vi "Set Motor Outputs.vi"(11 "Updated Drive Metrics in":T1) -> (3 "Updated Drive Metrics out":T1)   [LabVIEW 2014]
uses:
  Drive Train Metrics.ctl
  CmdFlag.ctl
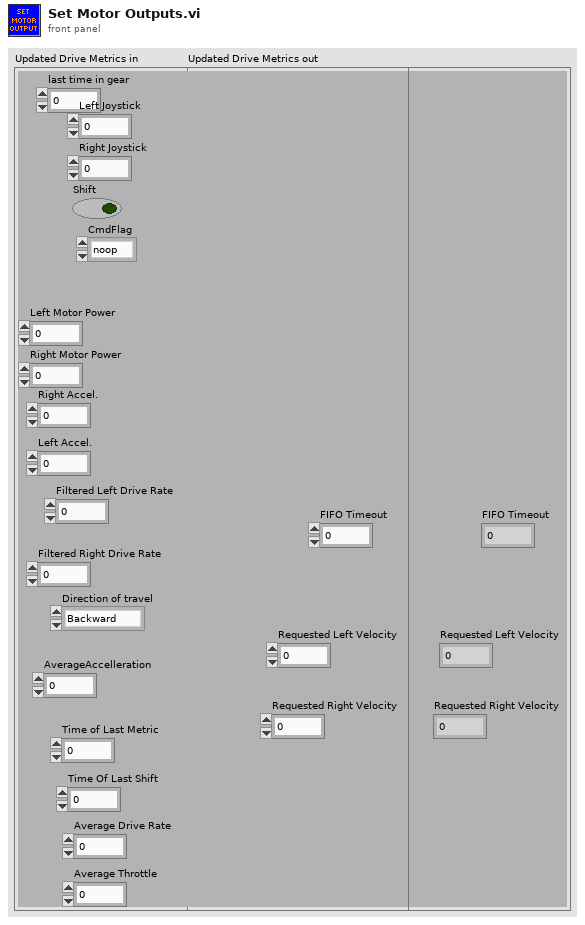
[diagram p1: front panel]
types:
  T1 = typedef "Drive Train Metrics.ctl" = cluster{"last time in gear":u32, "Shift":bool, "Right Joystick":dbl, "Left Joystick":dbl, "CmdFlag":T2, "Right Motor Power":dbl, "Left Motor Power":dbl, "Right Accel.":dbl, "Left Accel.":dbl, "Filtered Left Drive Rate":dbl, "Filtered Right Drive Rate":dbl, "Direction of travel":enum16{"Backward", "Forward", "Spin"}, "AverageAccelleration":dbl, "Time of Last Metric":u32, "Time Of Last Shift":dbl, "Average Drive Rate":dbl, "Average Throttle":dbl, "FIFO Timeout":i32, "Requested Left Velocity":dbl, "Requested Right Velocity":dbl}
  T2 = typedef "CmdFlag.ctl" = enum16{"noop", "suspend", "resume"}
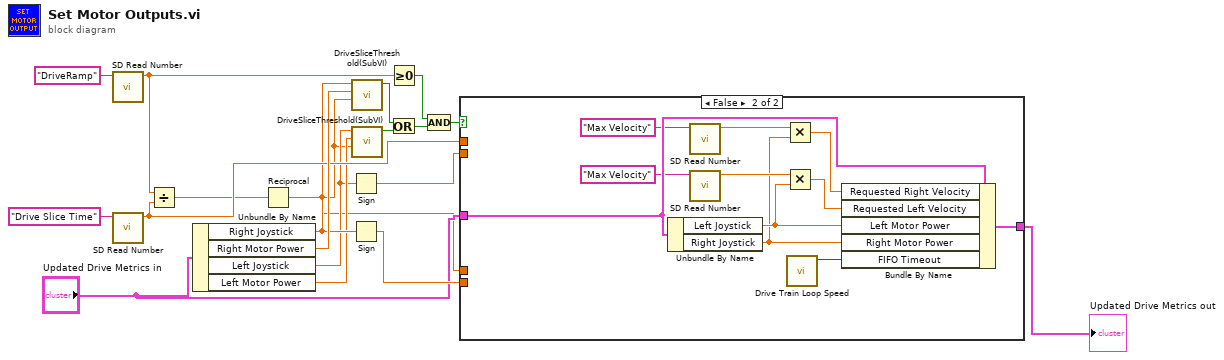
[diagram p0: block diagram]
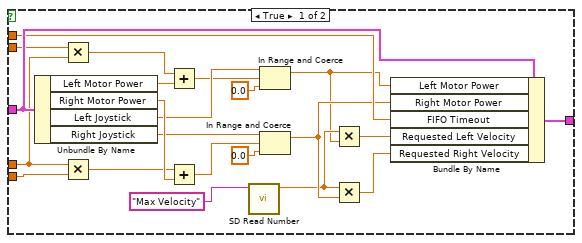
[diagram p2: hidden frame]
diagram:
  n1 = call <vilib>:"SD Read Number.vi"("Name"="DriveRamp") -> ("Numeric"=w16:dbl)  [unwired: 8 in, 2 out]
  n2 = call <vilib>:"SD Read Number.vi"("Name"="Drive Slice Time") -> ("Numeric"=w12:dbl)  [unwired: 8 in, 2 out]
  n3 = Divide(x=w16, y=w12) -> (x/y=w11:dbl)
  n4 = Unbundle By Name("Updated Drive Metrics in") -> ("Right Joystick"=w8:dbl, "Right Motor Power"=w15:dbl, "Left Joystick"=w3:dbl, "Left Motor Power"=w4:dbl)
  n5 = Reciprocal(x=w11) -> (1/x=w2:dbl)
  n6 = Sign(1:w3) -> (0:w6:dbl)
  n7 = Sign(1:w8) -> (0:w7:dbl)
  n8 = call "DriveSliceThreshold(SubVI).vi"("RampValue"=w2, "Motor Power"=w15, "Joystick"=w8) -> ("Boolean"=w9:bool)  [unwired: 8 in]
  n9 = call "DriveSliceThreshold(SubVI).vi"("RampValue"=w2, "Motor Power"=w4, "Joystick"=w3) -> ("Boolean"=w1:bool)  [unwired: 8 in]
  n10 = Greater Or Equal To 0?(x=w16) -> (x >= 0?=w18:bool)
  n11 = Or(x=w9, y=w1) -> (x .or. y?=w10:bool)
  n12 = Compound Arithmetic op=AND(w18, w10) -> (w14:bool)
  n13 = case shown="False" w14 {
    tunnel: "Updated Drive Metrics in" -> [w41 w52]
    tunnel: [w40 w51] -> w13
    tunnel: w12 -> [w39 _]
    tunnel: w2 -> [w33 _]
    tunnel: w7 -> [w36 _]
    tunnel: w6 -> [w34 _]
    frame True {
      n14 = Unbundle By Name(w41) -> ("Left Motor Power"=w38:dbl, "Right Motor Power"=w37:dbl, "Left Joystick"=w30:dbl, "Right Joystick"=w26:dbl)
      n15 = Multiply(x=w34, y=w33) -> (x*y=w32:dbl)
      n16 = Multiply(x=w33, y=w36) -> (x*y=w35:dbl)
      n17 = Add(x=w32, y=w38) -> (x+y=w29:dbl)
      n18 = Add(x=w35, y=w37) -> (x+y=w27:dbl)
      n19 = call <vilib>:"SD Read Number.vi"("Name"="Max Velocity") -> ("Numeric"=w22:dbl)  [unwired: 8 in, 2 out]
      n20 = In Range and Coerce(upper limit=w30, x=w29, lower limit=0.0) -> (coerced(x)=w21:dbl)  [unwired: 1 out]
      n21 = In Range and Coerce(upper limit=w26, x=w27, lower limit=0.0) -> (coerced(x)=w24:dbl)  [unwired: 1 out]
      n22 = Multiply(x=w22, y=w21) -> (x*y=w20:dbl)
      n23 = Multiply(x=w22, y=w24) -> (x*y=w23:dbl)
      n24 = Bundle By Name(cluster=w41, "Left Motor Power"=w21, "Right Motor Power"=w24, "FIFO Timeout"=w39, "Requested Left Velocity"=w20, "Requested Right Velocity"=w23) -> (w40:T1)
    }
    frame False {
      n25 = Unbundle By Name(w52) -> ("Left Joystick"=w48:dbl, "Right Joystick"=w42:dbl)
      n26 = call <vilib>:"SD Read Number.vi"("Name"="Max Velocity") -> ("Numeric"=w44:dbl)  [unwired: 8 in, 2 out]
      n27 = call <vilib>:"SD Read Number.vi"("Name"="Max Velocity") -> ("Numeric"=w46:dbl)  [unwired: 8 in, 2 out]
      n28 = Multiply(x=w44, y=w42) -> (x*y=w43:dbl)
      n29 = Multiply(x=w46, y=w48) -> (x*y=w47:dbl)
      n30 = call "Drive Train Loop Speed.vi"() -> ("FIFO Timeout"=w50:i32)  [unwired: 11 in]
      n31 = Bundle By Name(cluster=w52, "Requested Right Velocity"=w43, "Requested Left Velocity"=w47, "Left Motor Power"=w48, "Right Motor Power"=w42, "FIFO Timeout"=w50) -> (w51:T1)
    }
  }
  "Updated Drive Metrics out" <- w13
